vi "mainSynchro_PIV_LAT.vi"() -> ()   [LabVIEW 2023]
uses:
  sousVis/configUtilisateur.ctl
  sousVis/customParam.ctl
  sousVis/configFPGA.ctl
  sousVis/defaultParam.ctl
  <vilib>/Instr/_visa.llb/VISA Configure Serial Port (Instr).vi
panel:
  in  "Port Com contrôleur":refnum<visa-resource-name>
  in  "customParam":T1={"CamDelayToOpen(µs)"=10, "FLWidth(µs)"=10, "QSWidth(µs)"=10, "DelayFL_QS (µs)"=180, "CamDelayToClose(µs)"=100, "CamPivExposure(µs)"=100}
  in  "Configuration contrôleur":T2={"Nombre de période"=0, "Fréquence "=10, "Nb pulse préchauffe laser"=0, "skip_frame_PIV"=0, "skip_frame_LAT"=0, "Time beetwen pulses (µs)"=10000, "Temps LAT (µs)"=20000, "Temps expo LAT (µs)"=10000, "action"=enum."PIV"}
  in  "StopPIV":bool
  in  "Play Button":bool
  out "XY Graph":cluster{cluster{"t_periode":i32, dbl}[]}[](graph)
  out "error out":errorcluster
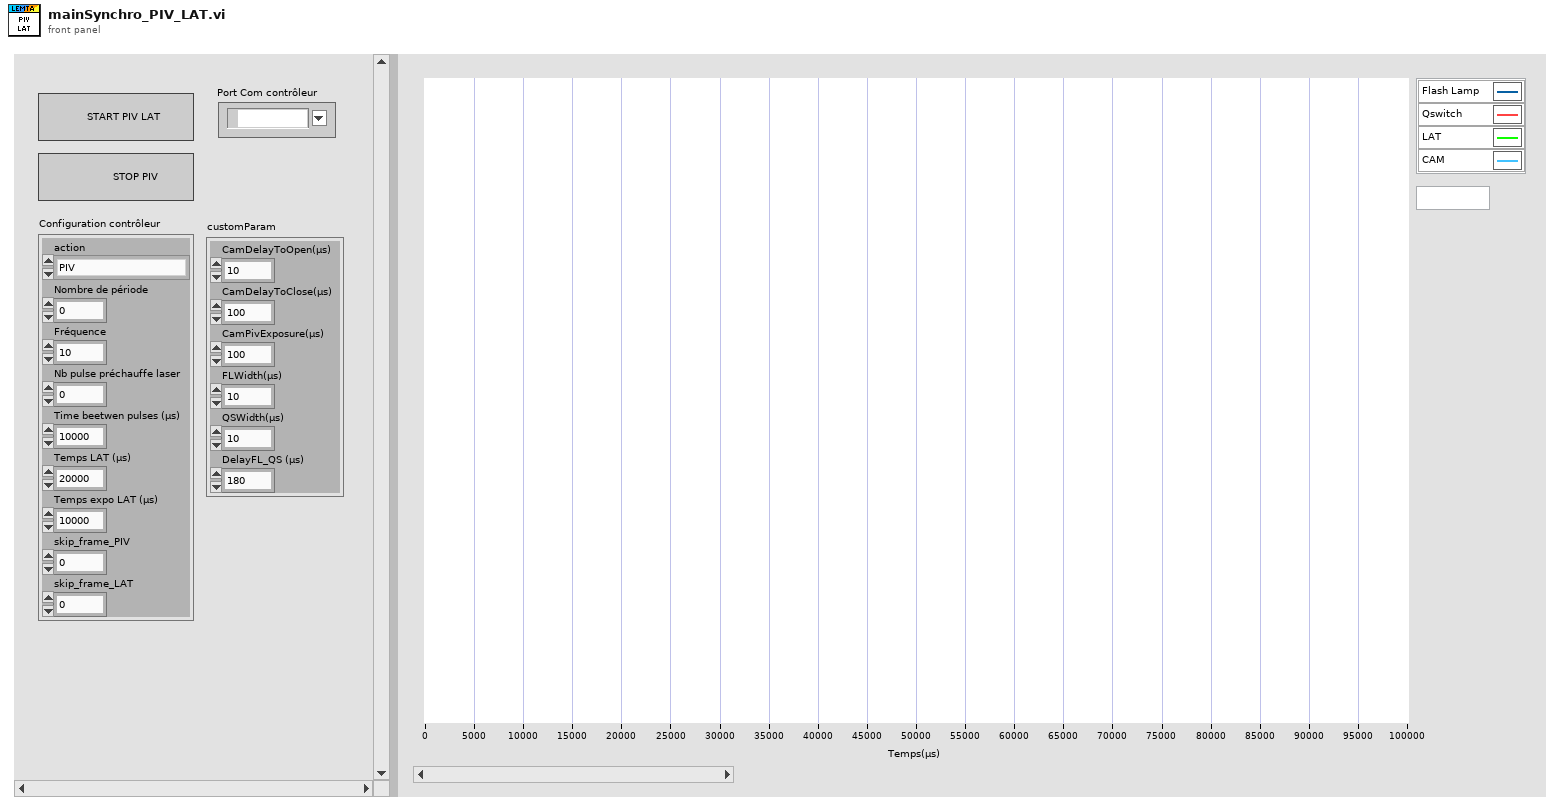
[diagram p1: front panel]
types:
  T1 = typedef "customParam.ctl" = cluster{"CamDelayToOpen(µs)":u32, "FLWidth(µs)":u32, "QSWidth(µs)":u32, "DelayFL_QS (µs)":u32, "CamDelayToClose(µs)":u32, "CamPivExposure(µs)":u32}
  T2 = typedef "configUtilisateur.ctl" = cluster{"Nombre de période":u16, "Fréquence ":u16, "Nb pulse préchauffe laser":u16, "skip_frame_PIV":u8, "skip_frame_LAT":u8, "Time beetwen pulses (µs)":u32, "Temps LAT (µs)":u32, "Temps expo LAT (µs)":u32, "action":enum8{"PIV", "PIV + LAT", "LAT"}}
  T3 = typedef "configFPGA.ctl" = cluster{"action":enum8{"PIV", "PIV + LAT", "LAT", "STOP"}, "nb_periodes":u16, "t_periode":u32, "nb_pulse_prechauffe":u8, "nb_skip_frame_PIV":u8, "nb_skip_frame_LAT":u8, "t_FL1_start":u32, "t_FL1_stop":u32, "t_QS1_start":u32, "t_QS1_stop":u32, "t_FL2_start":u32, "t_FL2_stop":u32, "t_QS2_start":u32, "t_QS2_stop":u32, "t_LAT_start":u32, "t_LAT_stop":u32, "t_FRAME1_start":u32, "t_FRAME1_stop":u32, "t_FRAME2_start":u32, "t_FRAME2_stop":u32}
  T4 = typedef "defaultParam.ctl" = cluster{"customParam":T1, "Configuration":T2}
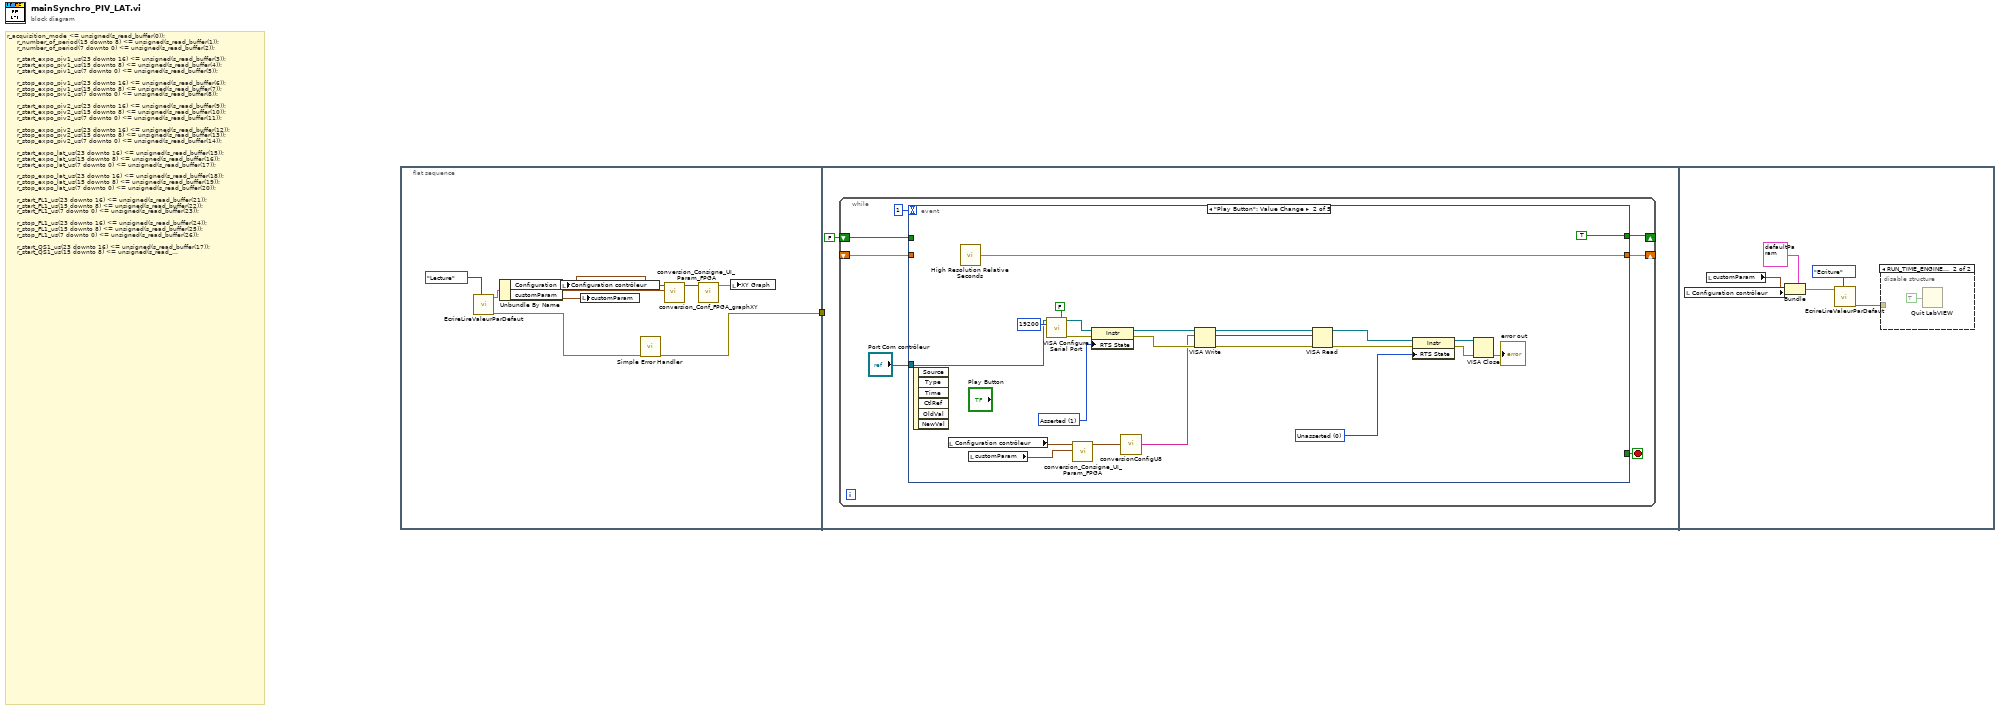
[diagram p0: block diagram]
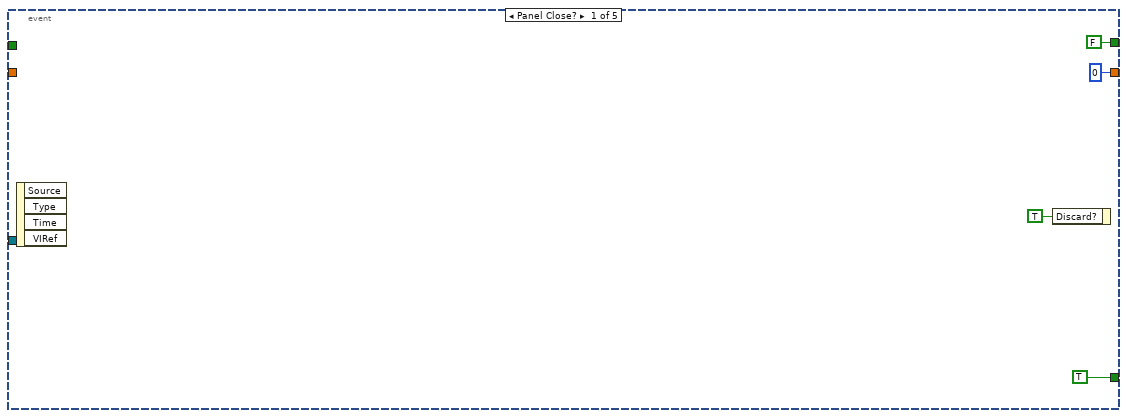
[diagram p2: hidden frame]
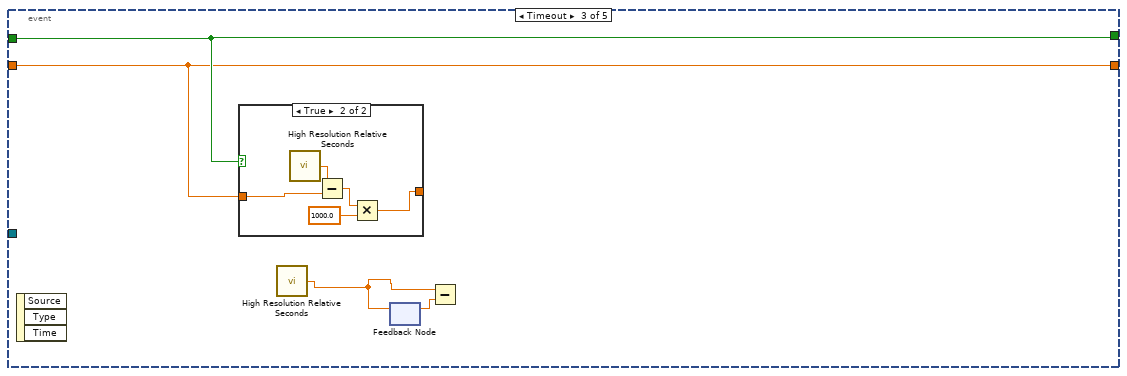
[diagram p3: hidden frame]
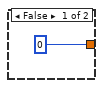
[diagram p4: hidden frame]
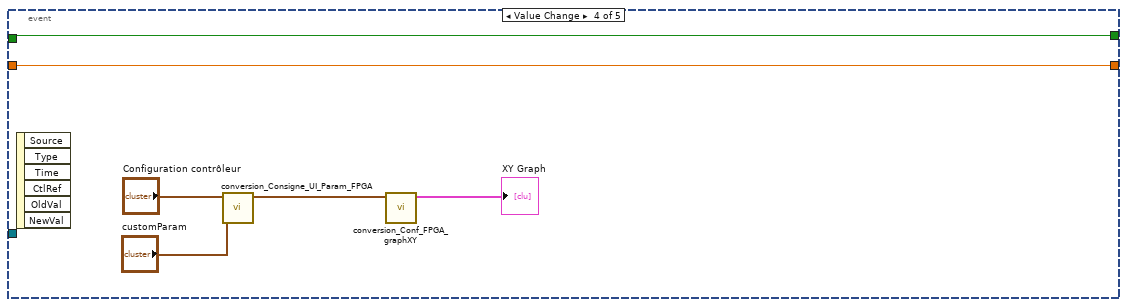
[diagram p5: hidden frame]
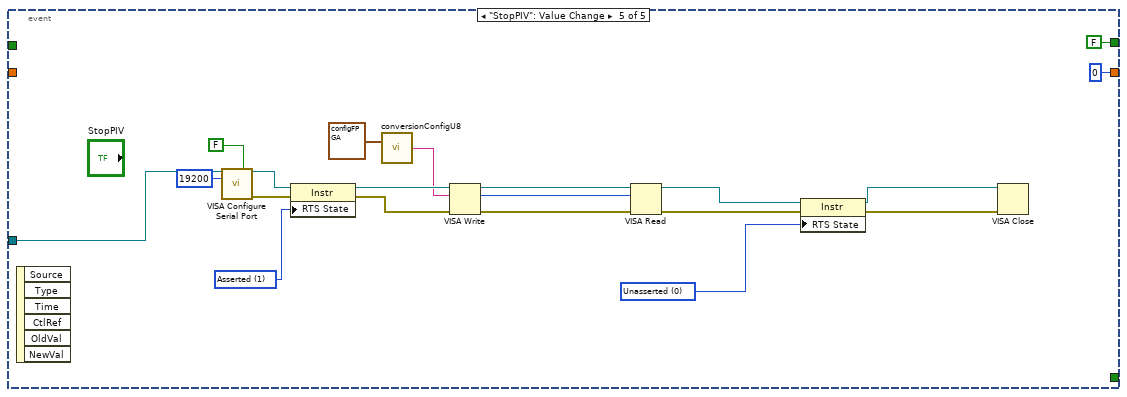
[diagram p6: hidden frame]
diagram:
  # "r_acquisition_mode <= unsigned(s_read_buffer(0));\n     r_number_of_period(15 downto 8) <= unsigned(s_read_buffer(1));\n\t\t\t\t\tr_number_of_period(7 downto 0) <= unsigned(s_read_buffer(2));\n\t\t\t\t\t\n\t\t\t\t\tr_start_expo_piv1_us(23 downto 16) <= unsigned(s_read_buffer(3));\n\t\t\t\t\tr_start_expo_piv1_us(15 downto 8) <= unsigned(s_read_buffer(4));\n\t\t\t\t\tr_start_expo_piv1_us(7 downto 0) <= unsigned(s_read_buffer(5));\n\t\t\t\t\t\n\t\t\t\t\tr_stop_expo_piv1_us(23 downto 16) <= unsigned(s_read_buffer(6));\n\t\t\t\t\tr_stop_expo_piv1_us(15 downto 8) <= unsigned(s_read_buffer(7));\n\t\t\t\t\tr_stop_expo_piv1_us(7 downto 0) <= unsigned(s_read_buffer(8));\n\t\t\t\t\t\n\t\t\t\t\tr_start_expo_piv2_us(23 downto 16) <= unsigned(s_read_buffer(9));\n\t\t\t\t\tr_start_expo_piv2_us(15 downto 8) <= unsigned(s_read_buffer(10));\n\t\t\t\t\tr_start_expo_piv2_us(7 downto 0) <= unsigned(s_read_buffer(11));\n\t\t\t\t\t\n\t\t\t\t\tr_stop_expo_piv2_us(23 downto 16) <= unsigned(s_read_buffer(12));\n\t\t\t\t\tr_stop_expo_piv2_us(15 downto 8) <= unsigned(s_read_buffer(13));\n\t\t\t\t\tr_stop_expo_piv2_us(7 downto 0) <= unsigned(s_read_buffer(14));\n\t\t\t\t\t\n\t\t\t\t\tr_start_expo_lat_us(23 downto 16) <= unsigned(s_read_buffer(15));\n\t\t\t\t\tr_start_expo_lat_us(15 downto 8) <= unsigned(s_read_buffer(16));\n\t\t\t\t\tr_start_expo_lat_us(7 downto 0) <= unsigned(s_read_buffer(17));\n\t\t\t\t\t\n\t\t\t\t\tr_stop_expo_lat_us(23 downto 16) <= unsigned(s_read_buffer(18));\n\t\t\t\t\tr_stop_expo_lat_us(15 downto 8) <= unsigned(s_read_buffer(19));\n\t\t\t\t\tr_stop_expo_lat_us(7 downto 0) <= unsigned(s_read_buffer(20));\n\t\t\t\t\t\n\t\t\t\t\tr_start_FL1_us(23 downto 16) <= unsigned(s_read_buffer(21));\n\t\t\t\t\tr_start_FL1_us(15 downto 8) <= unsigned(s_read_buffer(22));\n\t\t\t\t\tr_start_FL1_us(7 downto 0) <= unsigned(s_read_buffer(23));\n\t\t\t\t\t\n\t\t\t\t\tr_stop_FL1_us(23 downto 16) <= unsigned(s_read_buffer(24));\n\t\t\t\t\tr_stop_FL1_us(15 downto 8) <= unsigned(s_read_buffer(25));\n\t\t\t\t\tr_stop_FL1_us(7 downto 0) <= unsigned(s_read_buffer(26));\n\t\t\t\t\t\n\t\t\t\t\tr_start_QS1_us(23 downto 16) <= unsigned(s_read_buffer(17));\n\t\t\t\t\tr_start_QS1_us(15 downto 8) <= unsigned(s_read_buffer(28));\n\t\t\t\t\tr_start_QS1_us(7 downto 0) <= unsigned(s_read_buffer(29));\n\t\t\t\t\t\n\t\t\t\t\tr_stop_QS1_us(23 downto 16) <= unsigned(s_read_buffer(30));\n\t\t\t\t\tr_stop_QS1_us(15 downto 8) <= unsigned(s_read_buffer(31));\n\t\t\t\t\tr_stop_QS1_us(7 downto 0) <= unsigned(s_read_buffer(32));\n\t\t\t\t\t\n\t\t\t\t\tr_start_FL2_us(23 downto 16) <= unsigned(s_read_buffer(33));\n\t\t\t\t\tr_start_FL2_us(15 downto 8) <= unsigned(s_read_buffer(34));\n\t\t\t\t\tr_start_FL2_us(7 downto 0) <= unsigned(s_read_buffer(35));\n\t\t\t\t\t\n\t\t\t\t\tr_stop_FL2_us(23 downto 16) <= unsigned(s_read_buffer(36));\n\t\t\t\t\tr_stop_FL2_us(15 downto 8) <= unsigned(s_read_buffer(37));\n\t\t\t\t\tr_stop_FL2_us(7 downto 0) <= unsigned(s_read_buffer(38));\n\t\t\t\t\t\n\t\t\t\t\tr_start_QS2_us(23 downto 16) <= unsigned(s_read_buffer(39));\n\t\t\t\t\tr_start_QS2_us(15 downto 8) <= unsigned(s_read_buffer(40));\n\t\t\t\t\tr_start_QS2_us(7 downto 0) <= unsigned(s_read_buffer(41));\n\t\t\t\t\t\n\t\t\t\t\tr_stop_QS2_us(23 downto 16) <= unsigned(s_read_buffer(42));\n\t\t\t\t\tr_stop_QS2_us(15 downto 8) <= unsigned(s_read_buffer(43));\n\t\t\t\t\tr_stop_QS2_us(7 downto 0) <= unsigned(s_read_buffer(44));\n\t\t\t\t\t\n\t\t\t\t\tw_i_period_us(23 downto 16) <= unsigned(s_read_buffer(45));\n\t\t\t\t\tw_i_period_us(15 downto 8) <= unsigned(s_read_buffer(46));\n\t\t\t\t\tw_i_period_us(7 downto 0) <= unsigned(s_read_buffer(47));\n\t\t\t\t\t\n\t\t\t\t\tr_number_pulse_heat_laser(7 downto 0) <= unsigned(s_read_buffer(48));\n\t\t\t\t\t\n\t\t\t\t\tr_PIV_skip_frames(7 downto 0) <= unsigned(s_read_buffer(49));\n\t\t\t\t\t\n\t\t\t\t\tr_LAT_skip_frames(7 downto 0) <= unsigned(s_read_buffer(50));"
  n1 = flat-sequence {
    tunnel: [w2] -> w1
    tunnel: w1 -> [_]
    frame #0 {
      n2 = call "EcrireLireValeurParDefaut.vi"("Lecture/Ecriture"=enum32{"Lecture", "Ecriture"}."Lecture") -> ("error out"=w3:errorcluster, "defParametersOUT"=w8:T4)  [unwired: 8 in, 1 out]
      n3 = Unbundle By Name(w8) -> ("Configuration"=w7:T2, "customParam"=w6:T1)
      n4 = local write "Configuration contrôleur"(w7) -> ()
      n5 = local write "customParam"(w6) -> ()
      n6 = call <vilib>:"Simple Error Handler.vi"("error in (no error)"=w3) -> ("error out"=w2:errorcluster)  [unwired: 4 in, 4 out]
      n7 = call "conversion_Consigne_UI_Param_FPGA.vi"("customParam"=w6, "Config UI"=w7) -> ("Config FPGA"=w5:T3)  [unwired: 9 in]
      n8 = call "conversion_Conf_FPGA_graphXY.vi"("Config FPGA"=w5) -> ("appended array"=w4:cluster{cluster{"t_periode":i32, dbl}[]}[])  [unwired: 10 in]
      n9 = local write "XY Graph"(w4) -> ()
    }
    frame #1 {
      n10 = while {
        shift-right: [w14] -> _
        shift-left: _ -> [w11]
        shift-right: [w13] -> _
        shift-left: FALSE -> [w12]
        stop <- w17 stop-if-true
        n11 = event shown="[1] \"Play Button\": Value Change" {
          selector: _ -> [_ _ _ _ _]
          dyn-events: _ -> [_ _ _ _ _]
          timeout: 1 -> [_ _ _ _ _]
          tunnel: [TRUE _ _ _ _] -> w17
          tunnel: "Port Com contrôleur" -> [_ w29 _ _ w66]
          tunnel: [u32 0 ("millisecond timer value") w23 w47 w56 u32 0 ("millisecond timer value")] -> w14
          tunnel: [FALSE TRUE w48 w55 FALSE] -> w13
          tunnel: w12 -> [_ _ w48 w55 _]
          tunnel: w11 -> [_ _ w47 w56 _]
          event Panel Close? {
            n12 = event-data() -> ()  [unwired: 1 in, 4 out]
            n13 = event-data("Discard?"=TRUE) -> ()  [unwired: 1 in, 1 out]
          }
          event "Play Button": Value Change {
            w37 = i16 0 items=["Unknown"=-1, "Unasserted"=0, "Asserted"=1] ("Serial Settings:Modem Line Settings:Line RTS State")
            w43 = i16 1 items=["Unknown"=-1, "Unasserted"=0, "Asserted"=1] ("Serial Settings:Modem Line Settings:Line RTS State")
            n14 = event-data() -> ()  [unwired: 1 in, 6 out]
            n15 = local read "Configuration contrôleur"() -> (w26:T2)
            n16 = call <vilib>:"High Resolution Relative Seconds.vi"() -> ("relative seconds"=w23:dbl)
            n17 = local read "customParam"() -> (w25:T1)
            n18 = call-poly "VISA Configure Serial Port"("VISA resource name"=w29, "Enable Termination\nChar (T)"=FALSE ("Enable Termination\nChar (T)"), "baud rate (9600)"=u32 19200) -> ("VISA resource name out"=w42:refnum<visa-resource-name>, "error out"=w41:errorcluster)  [unwired: 11 in]
            n19 = call "conversion_Consigne_UI_Param_FPGA.vi"("customParam"=w25, "Config UI"=w26) -> ("Config FPGA"=w27:T3)  [unwired: 9 in]
            n20 = property class="Instr"(reference=w42, error in=w41, "RTS State"=w43) -> (reference out=w40:refnum<visa-resource-name>, error out=w39:errorcluster)
            n21 = call "conversionConfigU8.vi"("Config"=w27) -> ("TrameConsigne"=w22:string)
            n22 = VISA Write(VISA resource name=w40, write buffer=w22, error in (no error)=w39) -> (VISA resource name out=w35:refnum<visa-resource-name>, return count=w36:u32, error out=w28:errorcluster)
            n23 = VISA Read(VISA resource name=w35, byte count=w36, error in (no error)=w28) -> (VISA resource name out=w33:refnum<visa-resource-name>, error out=w34:errorcluster)  [unwired: 2 out]
            n24 = property class="Instr"(reference=w33, error in=w34, "RTS State"=w37) -> (reference out=w32:refnum<visa-resource-name>, error out=w31:errorcluster)
            n25 = VISA Close(VISA resource name=w32, error in (no error)=w31) -> (error out=→"error out":errorcluster)
          }
          event Timeout {
            n26 = event-data() -> ()  [unwired: 1 in, 3 out]
            n27 = case shown="True" w48 {
              tunnel: w47 -> [_ w54]
              tunnel: [u32 0 w51] -> _
              frame False {
              }
              frame True {
                n28 = call <vilib>:"High Resolution Relative Seconds.vi"() -> ("relative seconds"=w53:dbl)
                n29 = Subtract(x=w53, y=w54) -> (x-y=w52:dbl)
                n30 = Multiply(x=w52, y=1000.0) -> (x*y=w51:dbl)
              }
            }
            n31 = call <vilib>:"High Resolution Relative Seconds.vi"() -> ("relative seconds"=w45:dbl)
            n32 = feedback-in #1(w45) -> ()
            n33 = feedback #1() -> (w46:dbl)  [unwired: 1 in]
            n34 = Subtract(x=w45, y=w46) -> ()  [unwired: 1 out]
          }
          event Value Change {
            n35 = event-data() -> ()  [unwired: 1 in, 6 out]
            n36 = call "conversion_Consigne_UI_Param_FPGA.vi"("customParam"="customParam", "Config UI"="Configuration contrôleur") -> ("Config FPGA"=w59:T3)  [unwired: 9 in]
            n37 = call "conversion_Conf_FPGA_graphXY.vi"("Config FPGA"=w59) -> ("appended array"=→"XY Graph":cluster{cluster{"t_periode":i32, dbl}[]}[])  [unwired: 10 in]
          }
          event "StopPIV": Value Change {
            w74 = i16 0 items=["Unknown"=-1, "Unasserted"=0, "Asserted"=1] ("Serial Settings:Modem Line Settings:Line RTS State")
            w79 = i16 1 items=["Unknown"=-1, "Unasserted"=0, "Asserted"=1] ("Serial Settings:Modem Line Settings:Line RTS State")
            n38 = event-data() -> ()  [unwired: 1 in, 6 out]
            n39 = call-poly "VISA Configure Serial Port"("VISA resource name"=w66, "Enable Termination\nChar (T)"=FALSE ("Enable Termination\nChar (T)"), "baud rate (9600)"=u32 19200) -> ("VISA resource name out"=w78:refnum<visa-resource-name>, "error out"=w77:errorcluster)  [unwired: 11 in]
            n40 = property class="Instr"(reference=w78, error in=w77, "RTS State"=w79) -> (reference out=w76:refnum<visa-resource-name>, error out=w75:errorcluster)
            n41 = call "conversionConfigU8.vi"("Config"=T3 {"action"=enum."STOP", "nb_periodes"=0, "t_periode"=500000, "nb_pulse_prechauffe"=0, "nb_skip_frame_PIV"=0, "nb_skip_frame_LAT"=2, "t_FL1_start"=0, "t_FL1_stop"=100000, "t_QS1_start"=50000, "t_QS1_stop"=100000, "t_FL2_start"=100000, "t_FL2_stop"=200000, "t_QS2_start"=150000, "t_QS2_stop"=200000, "t_LAT_start"=300000, "t_LAT_stop"=400000, "t_FRAME1_start"=0, "t_FRAME1_stop"=100000, "t_FRAME2_start"=100000, "t_FRAME2_stop"=200000}) -> ("TrameConsigne"=w65:string)
            n42 = VISA Write(VISA resource name=w76, write buffer=w65, error in (no error)=w75) -> (VISA resource name out=w72:refnum<visa-resource-name>, return count=w73:u32, error out=w64:errorcluster)
            n43 = VISA Read(VISA resource name=w72, byte count=w73, error in (no error)=w64) -> (VISA resource name out=w70:refnum<visa-resource-name>, error out=w71:errorcluster)  [unwired: 2 out]
            n44 = property class="Instr"(reference=w70, error in=w71, "RTS State"=w74) -> (reference out=w69:refnum<visa-resource-name>, error out=w68:errorcluster)
            n45 = VISA Close(VISA resource name=w69, error in (no error)=w68) -> ()  [unwired: 1 out]
          }
        }
      }
    }
    frame #2 {
      n46 = local read "Configuration contrôleur"() -> (w83:T2)
      n47 = local read "customParam"() -> (w84:T1)
      n48 = Bundle(cluster=T4 {"customParam"={"CamDelayToOpen(µs)"=10, "FLWidth(µs)"=10, "QSWidth(µs)"=10, "DelayFL_QS (µs)"=180, "CamDelayToClose(µs)"=100, "CamPivExposure(µs)"=100}, "Configuration"={"Nombre de période"=2, "Fréquence "=0, "Nb pulse préchauffe laser"=41248, "skip_frame_PIV"=0, "skip_frame_LAT"=0, "Time beetwen pulses (µs)"=2, "Temps LAT (µs)"=0, "Temps expo LAT (µs)"=100000, "action"=enum."PIV + LAT"}} ("defParametersIN"), "customParam"=w84, "Configuration"=w83) -> (w82:T4)
      n49 = call "EcrireLireValeurParDefaut.vi"("Lecture/Ecriture"=enum32{"Lecture", "Ecriture"}."Ecriture", "defParametersIN"=w82) -> ("error out"=w81:errorcluster)  [unwired: 7 in, 2 out]
      n50 = disable-structure shown="RUN_TIME_ENGINE==True" {
        disable-tunnel: w81 -> [_ _]
        frame condition #0 (active) {
        }
        frame condition #1 {
          n51 = Quit LabVIEW(quit? (T)=TRUE) -> ()
        }
      }
    }
  }
